vi "Clear Trigger Event Detector.vi"(8 "error in (no error)":errorcluster, 9 "Trigger Number (1)":i32=1, 10 "Trigger Type (5: Trigger Generator)":i32(ring)=5 items=["Digital IO", "Blender", "Timer", "TSP Link", "LAN", "Trigger Generator "], 11 "VISA resource name":refnum<visa-resource-name>) -> (0 "error out":errorcluster, 3 "VISA resource name out":refnum<visa-resource-name>)   [LabVIEW 2017, in "Keithley 2600 Series.lvlib"]
doc: "Clears the trigger event detector and discards the history of command interface trigger events."
uses:
  <instrlib>/Keithley 2600 Series/Keithley 2600 Series.lvlib
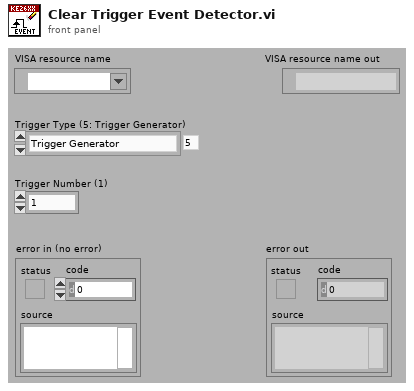
[diagram p1: front panel]
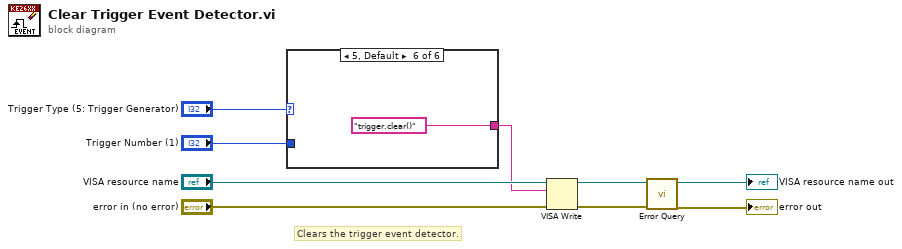
[diagram p0: block diagram]
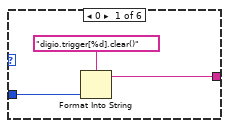
[diagram p2: hidden frame]
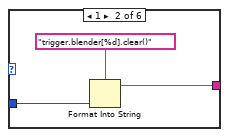
[diagram p3: hidden frame]
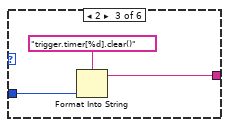
[diagram p4: hidden frame]
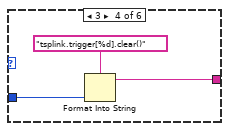
[diagram p5: hidden frame]
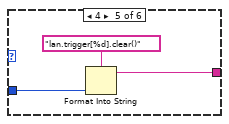
[diagram p6: hidden frame]
diagram:
  # "Clears the trigger event detector."
  n1 = case shown="5, Default" "Trigger Type (5: Trigger Generator)" {
    tunnel: "Trigger Number (1)" -> [w10 w14 w17 w20 w23 _]
    tunnel: [w11 w13 w16 w19 w22 "trigger.clear()"] -> w1
    frame 0 {
      n2 = Format Into String(format string="digio.trigger[%d].clear()", w10) -> (resulting string=w11:string)  [unwired: 2 in, 1 out]
    }
    frame 1 {
      n3 = Format Into String(format string="trigger.blender[%d].clear()", w14) -> (resulting string=w13:string)  [unwired: 2 in, 1 out]
    }
    frame 2 {
      n4 = Format Into String(format string="trigger.timer[%d].clear()", w17) -> (resulting string=w16:string)  [unwired: 2 in, 1 out]
    }
    frame 3 {
      n5 = Format Into String(format string="tsplink.trigger[%d].clear()", w20) -> (resulting string=w19:string)  [unwired: 2 in, 1 out]
    }
    frame 4 {
      n6 = Format Into String(format string="lan.trigger[%d].clear()", w23) -> (resulting string=w22:string)  [unwired: 2 in, 1 out]
    }
    frame 5, Default {
    }
  }
  n7 = VISA Write(VISA resource name="VISA resource name", write buffer=w1, error in (no error)="error in (no error)") -> (VISA resource name out=w7:refnum<visa-resource-name>, error out=w6:errorcluster)  [unwired: 1 out]
  n8 = call <instrlib>:"Error Query.vi"("error in (no error)"=w6, "VISA resource name"=w7) -> ("error out"=→"error out":errorcluster, "VISA resource name out"=→"VISA resource name out":refnum<visa-resource-name>)  [unwired: 6 in, 2 out]
